vi "EOL O'Scope Data.vi"(11 "station names":string[](array[string])) -> ()   [LabVIEW 2018]
uses:
  02.Type Def's/EOL Analog Input Control.ctl
panel:
  out "Current Max":sgl
  out "Last ATS":sgl
  out "Current":sgl
  out "ATS":sgl
  in  "station selector":u16(ring) items=["St0-InitATS", "", "", "", "", ""]
  in  "Color Box 16":u32(colorbox)=9567230
  in  "Color Box 15":u32(colorbox)=16711935
  in  "Analog Control 7":T1=enum."Motor Voltage"
  in  "Analog Control 6":T1=enum."ATS"
  in  "Analog Control 5":T1=enum."Motor Current"
  in  "Analog Control 4":T1=enum."Switch B"
  in  "Analog Control 3":T1=enum."Switch A"
  in  "Analog Control 2":T1=enum."Switch A"
  in  "Pause Data Collection":bool
  in  "Color Box 14":u32(colorbox)=15695616
  in  "Color Box 13":u32(colorbox)=1985280
  in  "Analog Control":T1
  in  "Color Box 10":u32(colorbox)=16860
  in  "Color Box 11":u32(colorbox)=16711680
  in  "Color Box 12":u32(colorbox)
  out "Audit Graph":sgl[][](graph)
  in  "Exit":bool
  # "O'Scope Data Display"
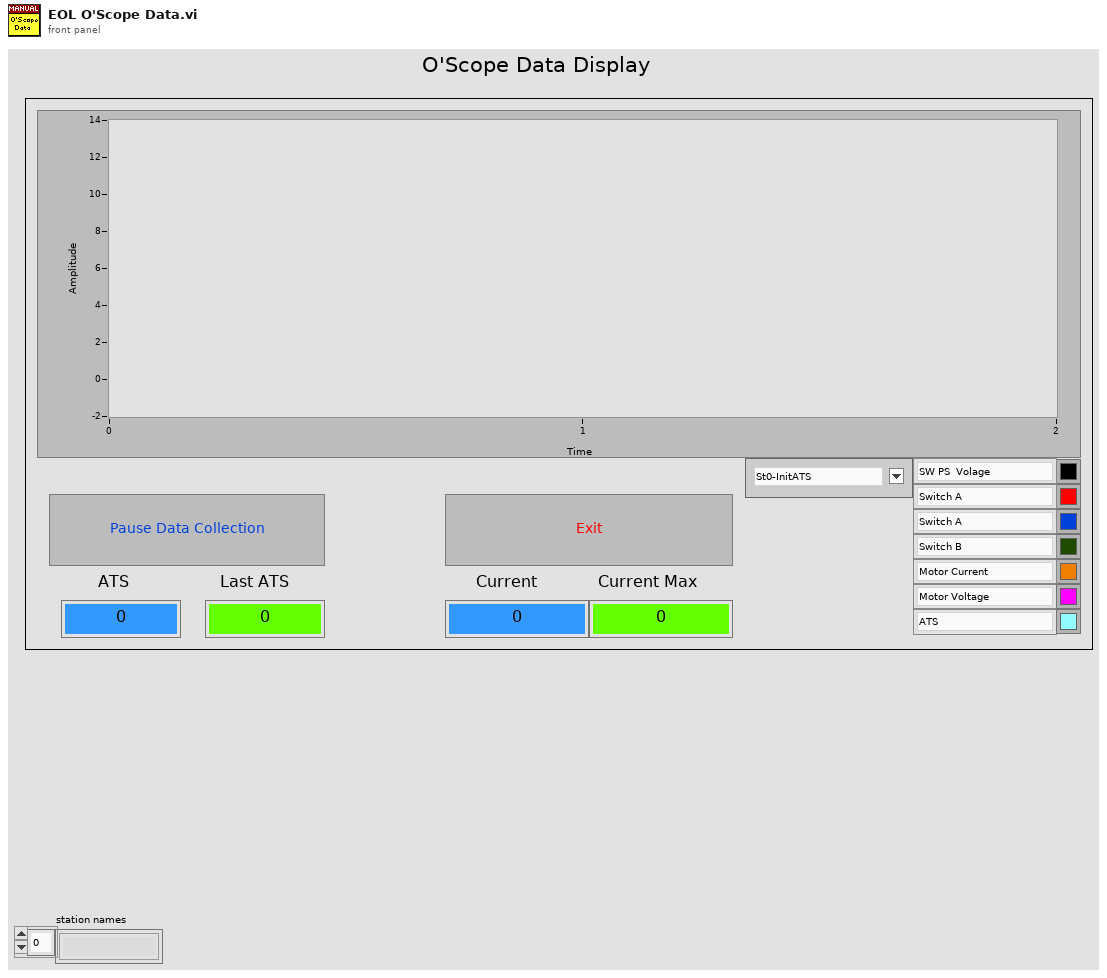
[diagram p1: front panel]
types:
  T1 = typedef "EOL Analog Input Control.ctl" = enum16{"SW PS  Volage", "Switch A", "Switch B", "Switch C", "Motor Voltage", "Motor Current", "ATS"}
  T2 = enum16{"SW PS Voltage", "SW IGN Bat", "Switch A", "Switch B", "Motor Voltage", "Motor Current", "SW LIN"}
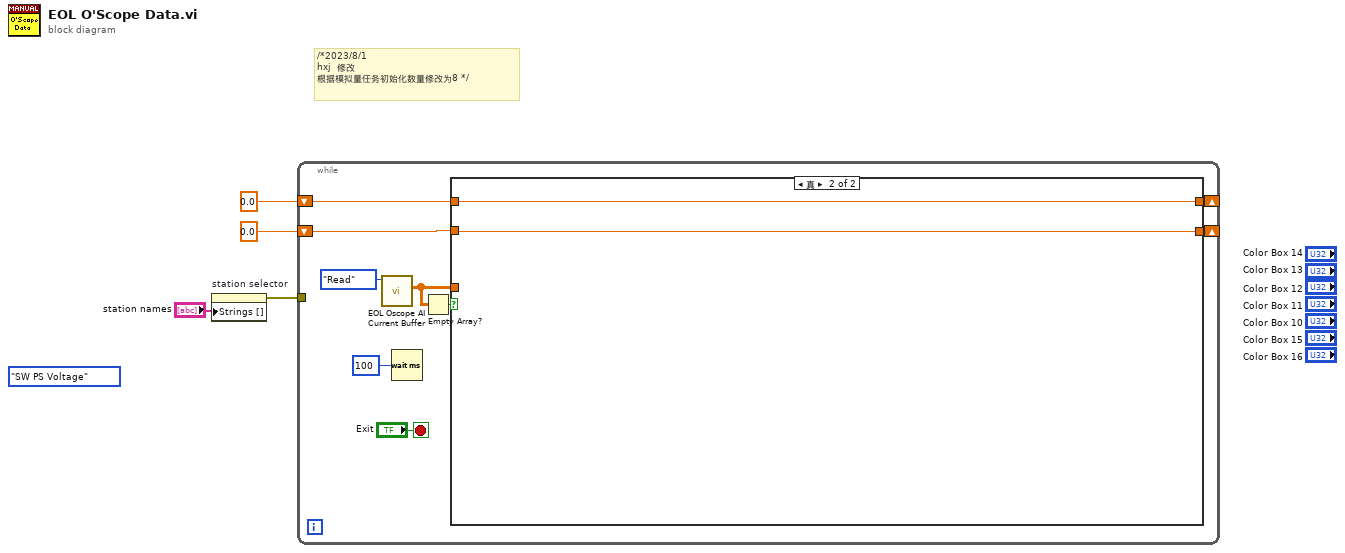
[diagram p0: block diagram]
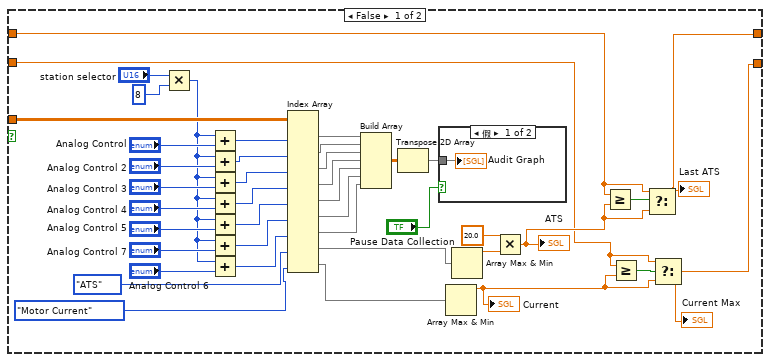
[diagram p2: hidden frame]
diagram:
  (unwired) T2."SW PS Voltage"
  # "/*2023/8/1\nhxj  修改\n根据模拟量任务初始化数量修改为8 */"
  n1 = property on="station selector" class="Ring (strict)"("Strings []"="station names") -> (error out=w3:errorcluster)  [unwired: 2 in, 1 out]
  n2 = while {
    tunnel: w3 -> [_]
    shift-right: [w7] -> _
    shift-left: sgl 0.0 ("x") -> [w8]
    shift-right: [w5] -> _
    shift-left: sgl 0.0 ("x") -> [w6]
    stop <- "Exit" stop-if-true
    n3 = call "EOL Oscope AI Current Buffer.vi"("Mode"=enum16{"Initialize", "Read", "Write"}."Read") -> ("Data Read (Ch-Ro, Samp-Col)"=w9:sgl[][])  [unwired: 10 in]
    n4 = Wait (ms)(milliseconds to wait=u32 100) -> ()  [unwired: 1 out]
    n5 = Empty Array?(array=w9) -> (empty?=w10:bool)
    n6 = case shown="真" w10 {
      tunnel: w9 -> [w55 _]
      tunnel: w8 -> [w20 w58]
      tunnel: [w18 w58] -> w7
      tunnel: w6 -> [w16 w57]
      tunnel: [w14 w57] -> w5
      frame False {
        n7 = Multiply(x="station selector", y=8) -> (x*y=w40:i32)
        n8 = Add(x=w40, y="Analog Control") -> (x+y=w35:i32)
        n9 = Add(x=w40, y="Analog Control 2") -> (x+y=w34:i32)
        n10 = Add(x=w40, y="Analog Control 3") -> (x+y=w33:i32)
        n11 = Add(x=w40, y="Analog Control 4") -> (x+y=w32:i32)
        n12 = Add(x=w40, y="Analog Control 5") -> (x+y=w31:i32)
        n13 = Add(x=w40, y="Analog Control 7") -> (x+y=w30:i32)
        n14 = Add(x=w40, y="Analog Control 6") -> (x+y=w29:i32)
        n15 = Index Array(array=w55, index (col) #1=w35, index (col) #2=w34, index (col) #3=w33, index (col) #4=w32, index (col) #5=w31, index (col) #6=w30, index (col) #7=w29, index (col) #8=EOL_Analog_Input_Control."ATS" ("Analog Control 6"), index (col) #9=EOL_Analog_Input_Control."Motor Current" ("Analog Control 6")) -> (element #1=w52:sgl[], element #2=w53:sgl[], element #3=w54:sgl[], element #4=w51:sgl[], element #5=w50:sgl[], element #6=w39:sgl[], element #7=w38:sgl[], element #8=w26:sgl[], element #9=w24:sgl[])  [unwired: 9 in]
        n16 = Build Array(w52, w53, w54, w51, w50, w39, w38) -> (w37:sgl[][])
        n17 = Transpose 2D Array(2D array=w37) -> (transposed array=w36:sgl[][])
        n18 = case shown="假" "Pause Data Collection" {
          tunnel: w36 -> [w56 _]
          frame False {
            "Audit Graph" <- w56
          }
          frame True {
          }
        }
        n19 = Array Max & Min(array=w24) -> (max value=w15:sgl)  [unwired: 3 out]
        "Current" <- w15
        n20 = Array Max & Min(array=w26) -> (max value=w23:sgl)  [unwired: 3 out]
        n21 = Multiply(x=sgl 20.0, y=w23) -> (x*y=w19:sgl)
        "ATS" <- w19
        n22 = Greater Or Equal?(x=w20, y=w19) -> (x >= y?=w21:bool)
        n23 = Greater Or Equal?(x=w16, y=w15) -> (x >= y?=w17:bool)
        n24 = Select(t=w20, s=w21, f=w19) -> (s? t:f=w18:sgl)
        "Last ATS" <- w18
        n25 = Select(t=w16, s=w17, f=w15) -> (s? t:f=w14:sgl)
        "Current Max" <- w14
      }
      frame True {
      }
    }
  }
